vi "SWERVE_GET_MAX.vi"() -> (1 "Max Rotational Vel (Rad/Sec)":dbl, 3 "Max Wheel Vel (Meter/Sec)":dbl)   [LabVIEW 2019]
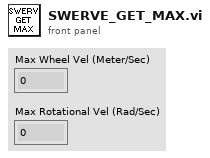
[diagram p1: front panel]
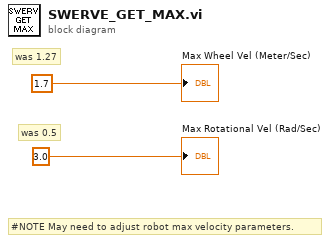
[diagram p0: block diagram]
diagram:
  # "#NOTE May need to adjust robot max velocity parameters."
  # "was 0.5"
  # "was 1.27"
  "Max Wheel Vel (Meter/Sec)" <- 1.7
  "Max Rotational Vel (Rad/Sec)" <- 3.0
